vi "Omron_COMM_Close.vi"(8 "error in":errorcluster, 11 "COM in":refnum<visa-resource-name>) -> (0 "error out":errorcluster)   [LabVIEW 2015]
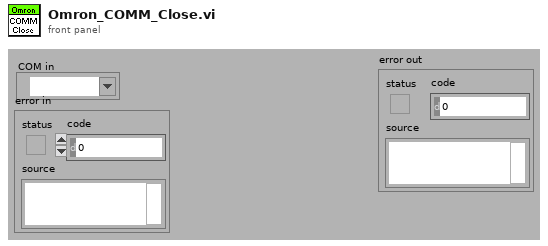
[diagram p1: front panel]
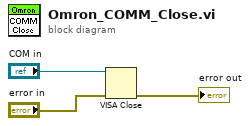
[diagram p0: block diagram]
diagram:
  n1 = VISA Close(VISA resource name="COM in", error in (no error)="error in") -> (error out=→"error out":errorcluster)
